vi "onCreateListener.vi"(6 "timeout (ms)":i32=100, 8 "error in (no error)":errorcluster, 10 "Configuration":refnum<class "Connection.TCP-TLS.lvclass">) -> (0 "error out":errorcluster, 3 "Listener":refnum<class "Connection.lvclass">)   [LabVIEW 2020, in "Connection.TCP-TLS.lvclass"]
uses:
  Connection.TCP-TLS.lvclass
  C:/Program Files (x86)/National Instruments/LabVIEW 2020/vi.lib/LabVIEW Open Source Project/MQTT Connection/MQTT_Connection/Connection/Connection.lvclass
  <vilib>/LabVIEW Open Source Project/MQTT Connection/MQTT_Connection/Connection/Connection.lvclass
  Connection.TCP-TLS.lvclass/Connection.TCP-TLS.ctl
  <vilib>/LabVIEW Open Source Project/MQTT TCP Connection/MQTT_TCP/Connection/TCPConnection.lvclass
  C:/Program Files (x86)/National Instruments/LabVIEW 2020/vi.lib/LabVIEW Open Source Project/MQTT TCP Connection/MQTT_TCP/Connection/TCPConnection.lvclass
  C:/Projects/LVOS/MQTT-Connection-TCP.TLS/source/Connection.SecuredTCP/Connection.TCP-TLS.lvclass
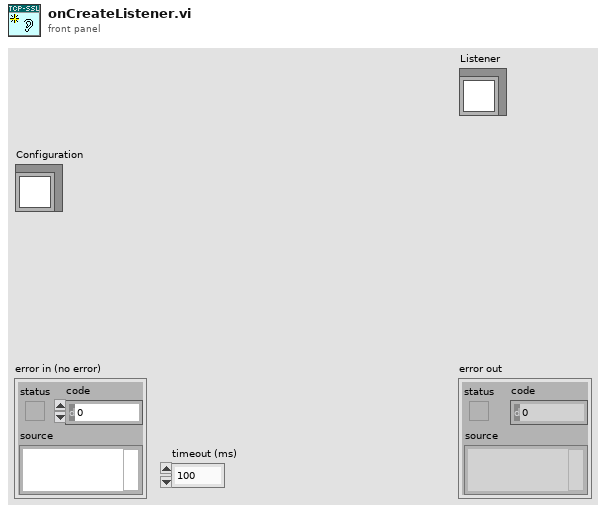
[diagram p1: front panel]
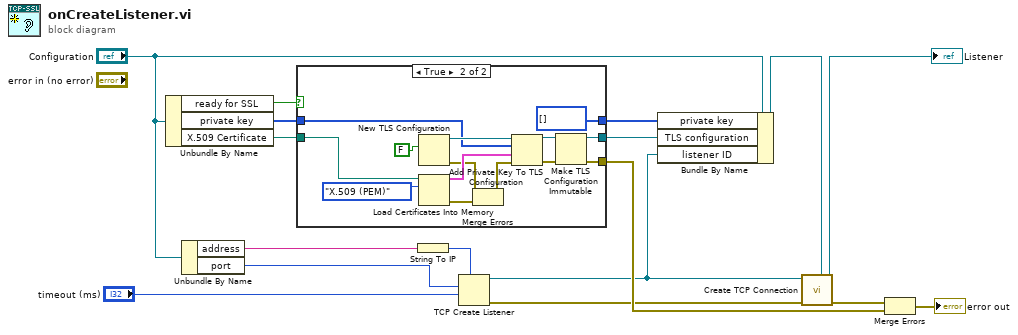
[diagram p0: block diagram]
diagram:
  n1 = Unbundle By Name("Configuration") -> ("ready for SSL"=w14:bool, "private key"=w12:u8[], "X.509 Certificate"=w13:path)
  n2 = Unbundle By Name("Configuration") -> ("address"=w15:string, "port"=w17:u16)
  n3 = case shown="True" w14 {
    tunnel: w13 -> [_ w26]
    tunnel: w12 -> [w18 w25]
    tunnel: [_ w24] -> w11
    tunnel: [_ w20] -> w10
    tunnel: [w18 u8[] [] ("private key")] -> w8
    frame False {
    }
    frame True {
      n4 = New TLS Configuration(10:FALSE ("load OS trusted CAs?")) -> (0:w22:errorcluster, 3:w31:refnum<k36>)  [unwired: 1 in]
      n5 = Load Certificates Into Memory(10:enum32{"X.509 (PEM)"}."X.509 (PEM)" ("format"), 11:w26) -> (0:w23:errorcluster, 3:w32:cluster{"certificate":u8[]}[])  [unwired: 1 in]
      n6 = Merge Errors(w22, w23) -> (w21:errorcluster)
      n7 = Add Private Key To TLS Configuration(8:w21, 9:w32, 10:w25, 11:w31) -> (0:w30:errorcluster, 3:w29:refnum<k36>)
      n8 = Make TLS Configuration Immutable(8:w30, 11:w29) -> (0:w20:errorcluster, 3:w24:refnum<k36>)
    }
  }
  n9 = String To IP(1:w15) -> (0:w6:u32)
  n10 = TCP Create Listener(7:w6, 9:"timeout (ms)", 10:w17) -> (0:w3:errorcluster, 3:w1:refnum<k5>)  [unwired: 2 in, 1 out]
  n11 = Bundle By Name(cluster="Configuration", "private key"=w8, "TLS configuration"=w11, "listener ID"=w1) -> (w5:refnum<class "Connection.TCP-TLS.lvclass">)
  n12 = call <vilib>:"Create TCP Connection.vi"("TCPConnection in"=w5, "error in (no error)"=w3, "connection ID"=w1) -> ("error out"=w2:errorcluster, "TCPConnection out"=→"Listener":refnum<class "Connection.TCP-TLS.lvclass">)  [unwired: 7 in]
  n13 = Merge Errors(w2, w10) -> (→"error out":errorcluster)
